vi "Connect List.vi"(8 "error in (no error)":errorcluster, 10 "Params":variant, 11 "PIPXI40 Switching in":refnum<class "PIPXI40 GP Switch.lvclass">) -> (0 "error out":errorcluster, 3 "PIPXI40 Switching out":refnum<class "PIPXI40 GP Switch.lvclass">)   [LabVIEW 2020, in "PIPXI40.lvlib" / "PIPXI40 GP Switch.lvclass"]
uses:
  PIPXI40 GP Switch.lvclass
  D:/WSGitHub/RTFWK/Realization/PIPXI40 Base/PIPXI40 Base.lvclass
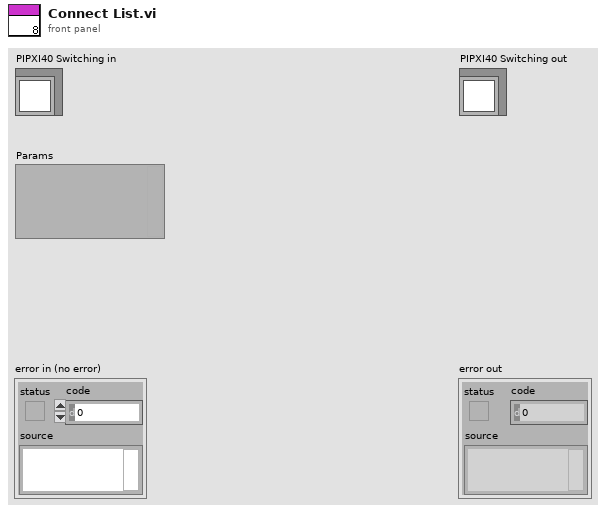
[diagram p1: front panel]
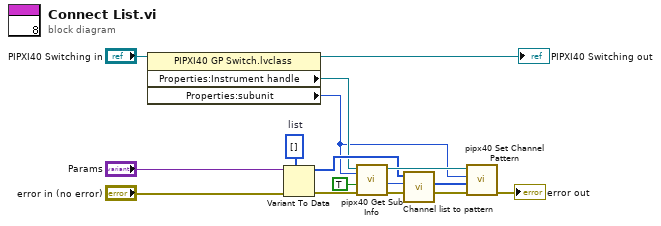
[diagram p0: block diagram]
diagram:
  w8 = i32[] []  # list
  n1 = property class="PIPXI40 GP Switch.lvclass"(reference="PIPXI40 Switching in") -> (reference out=→"PIPXI40 Switching out":refnum<class "PIPXI40 GP Switch.lvclass">, "Properties:Instrument handle"=w3:refnum<visa-resource-name>, "Properties:subunit"=w2:u32)  [unwired: 1 in, 1 out]
  n2 = Variant To Data(error in="error in (no error)", type=w8, Variant="Params") -> (data=w6:i32[], error out=w12:errorcluster)
  n3 = call <instrlib>:"pipx40 Get Sub Info.vi"("error in (no error)"=w12, "is output"=TRUE, "subunit number"=w2, "instrument handle"=w3) -> ("error out"=w11:errorcluster, "columns"=w10:u32, "instrument handle out"=w9:refnum<visa-resource-name>)  [unwired: 3 in, 2 out]
  n4 = call "Channel list to pattern.vi"("Outputs"=w10, "List"=w6) -> ("Pattern"=w5:u32[])  [unwired: 9 in]
  n5 = call <instrlib>:"pipx40 Set Channel Pattern.vi"("error in (no error)"=w11, "pattern"=w5, "subunit number"=w2, "instrument handle"=w9) -> ("error out"=→"error out":errorcluster)  [unwired: 6 in, 1 out]
